vi "BL_Disconnect.vi"(8 "error in (no error)":errorcluster, 11 "Potentiostat Galvanostat in":refnum<class "Potentiostat Galvanostat.lvclass">) -> (0 "error out":errorcluster, 3 "Potentiostat Galvanostat out":refnum<class "Potentiostat Galvanostat.lvclass">)   [LabVIEW 2018, in "Potentiostat Galvanostat.lvclass"]
uses:
  Potentiostat Galvanostat.lvclass
  Potentiostat Galvanostat.lvclass/Potentiostat Galvanostat.ctl
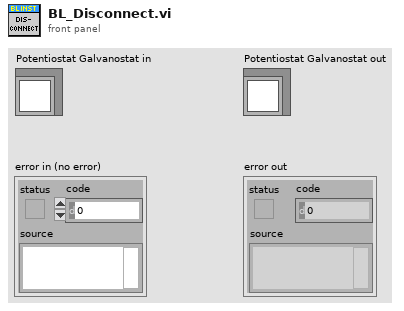
[diagram p1: front panel]
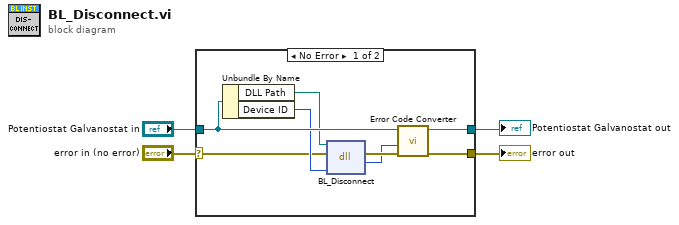
[diagram p0: block diagram]
diagram:
  n1 = case shown="No Error" "error in (no error)" {
    selector: "error in (no error)" -> [w5 w14]
    tunnel: "Potentiostat Galvanostat in" -> [w12 w13]
    tunnel: [w11 w13] -> w3
    tunnel: [w6 w14] -> w2
    frame No Error {
      n2 = Unbundle By Name(w12) -> ("DLL Path"=w10:path, "Device ID"=w7:i32)
      n3 = dll-call lib="C:/Projects/LabVIEW/BioLogic Instrument Driver/libs/EC-Lab Development Package/EClib.*" fn="BL_Disconnect"(path in=w10, error in=w5, "Device ID"=w7) -> (error out=w9:errorcluster, "Error Code"=w8:i32)  [unwired: 2 in, 1 out]
      n4 = call-dynamic "Error Code Converter.vi"("error in (no error)"=w9, "Error Code"=w8, "Potentiostat Galvanostat in"=w12) -> ("error out"=w6:errorcluster, "Potentiostat Galvanostat out"=w11:refnum<class "Potentiostat Galvanostat.lvclass">)  [unwired: 7 in]
    }
    frame Error {
    }
  }
  "error out" <- w2
  "Potentiostat Galvanostat out" <- w3
